vi "Page_Version_Initialize.vi"(6 "output cluster":T1, 8 "error in (no error)":errorcluster, 11 "Build in":refnum<class "AB_Build.lvclass">) -> (0 "error out":errorcluster, 3 "Build out":refnum<class "AB_Build.lvclass">)   [LabVIEW 2020, in "AB_Deployment.lvlib"]
uses:
  <vilib>/AppBuilder/AB_Classes/Deployment/AB_Deployment.lvlib
  <vilib>/AppBuilder/AB_Classes/Build/AB_Build.lvclass
  <resource>/Framework/Providers/Builds/AppBuilder/AB_UI_Page_Version_References.ctl
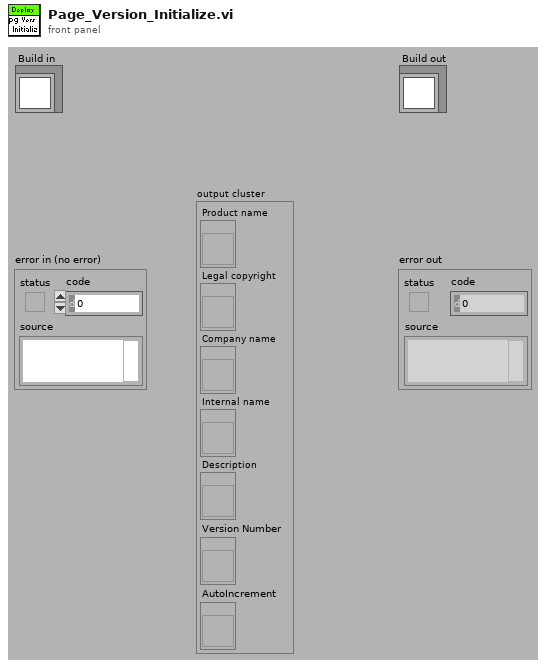
[diagram p1: front panel]
types:
  T1 = typedef "AB_UI_Page_Version_References.ctl" = cluster{"Product name":refnum<vi>, "Legal copyright":refnum<vi>, "Company name":refnum<vi>, "Internal name":refnum<vi>, "Description":refnum<vi>, "Version Number":refnum<vi>, "AutoIncrement":refnum<vi>}
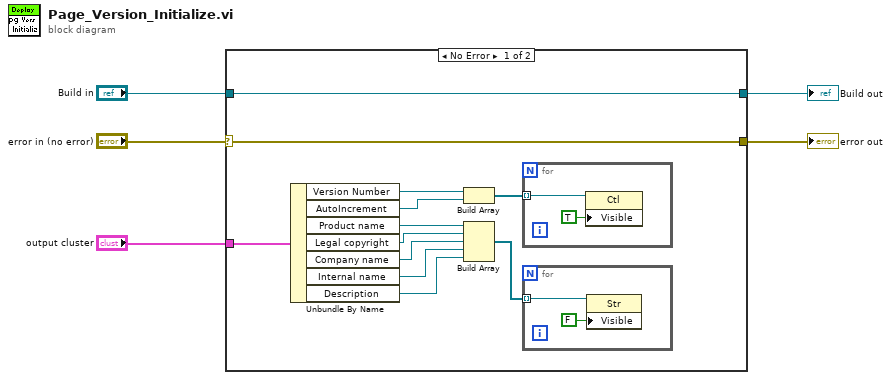
[diagram p0: block diagram]
diagram:
  n1 = case shown="No Error" "error in (no error)" {
    selector: "error in (no error)" -> [w7 w22]
    tunnel: "Build in" -> [w8 w23]
    tunnel: [w8 w23] -> w4
    tunnel: [w7 w22] -> w3
    tunnel: "output cluster" -> [w6 _]
    frame No Error {
      n2 = Unbundle By Name(w6) -> ("Version Number"=w17:refnum<vi>, "AutoIncrement"=w16:refnum<vi>, "Product name"=w14:refnum<vi>, "Legal copyright"=w13:refnum<vi>, "Company name"=w12:refnum<vi>, "Internal name"=w11:refnum<vi>, "Description"=w10:refnum<vi>)
      n3 = Build Array(w17, w16) -> (w15:refnum<vi>[])
      n4 = Build Array(w14, w13, w12, w11, w10) -> (w9:refnum<vi>[])
      n5 = for {
        tunnel: w15 -> [w21] mode=indexing
        n6 = property class="Ctl"(reference=w21, "Visible"=TRUE) -> ()  [unwired: 1 in, 2 out]
      }
      n7 = for {
        tunnel: w9 -> [w19] mode=indexing
        n8 = property class="Str"(reference=w19, "Visible"=FALSE) -> ()  [unwired: 1 in, 2 out]
      }
    }
    frame Error {
    }
  }
  "error out" <- w3
  "Build out" <- w4
